vi "HEWH Adjust Gas Energy at 23 hours.vi"(0 "Full Data w/o Information Header in":dbl[][](array[numeric]) format="%#_6f", 2 "Test Start Index  (Full Index)":i32, 3 "Energy (BTU) Index":i32, 5 "error in (no error)":errorcluster) -> (14 "Qf":dbl, 15 "Start Energy (BTU-Gas)":dbl format="%#_6f", 19 "error out":errorcluster)   [LabVIEW 2020]
panel:
  out "End Energy (BTU-Gas)":dbl format="%#_11f"
  out "23 Hour Index":i32
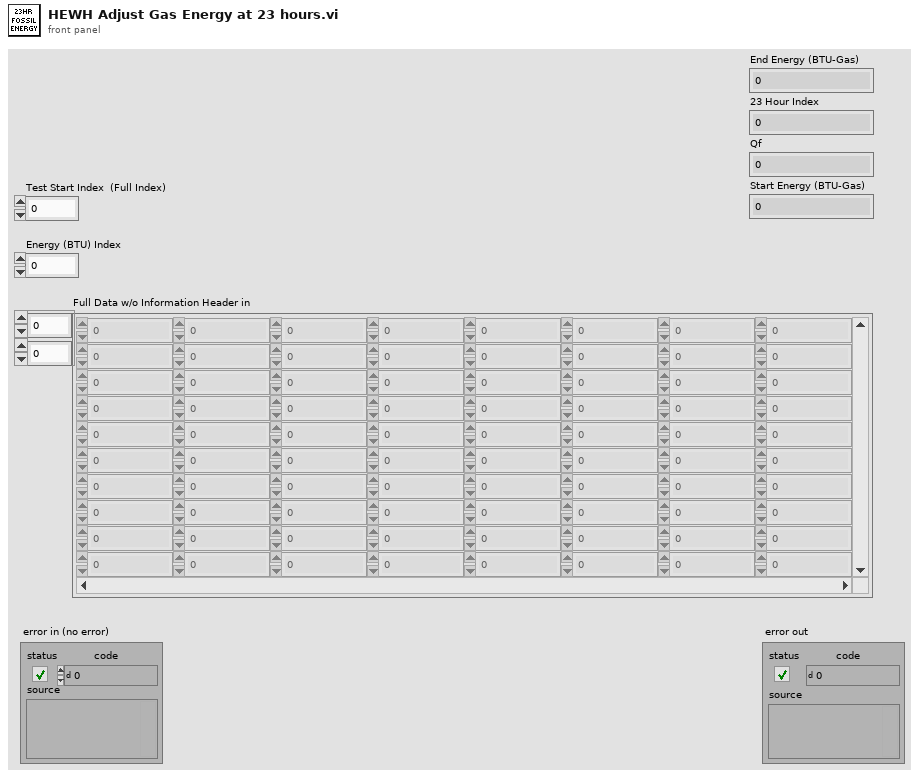
[diagram p1: front panel]
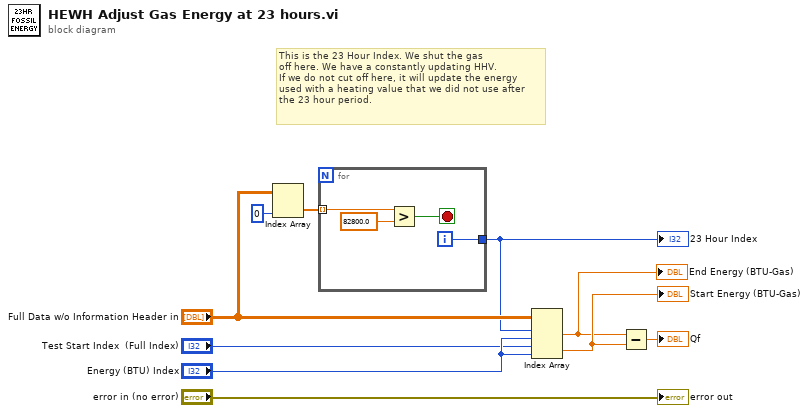
[diagram p0: block diagram]
diagram:
  # "This is the 23 Hour Index. We shut the gas\noff here. We have a constantly updating HHV. \nIf we do not cut off here, it will update the energy \nused with a heating value that we did not use after\nthe 23 hour period."
  n1 = Index Array(array="Full Data w/o Information Header in", index (col)=0 ("disabled index (col)")) -> (element=w2:dbl[])  [unwired: 1 in]
  n2 = for {
    tunnel: w2 -> [w14] mode=indexing
    tunnel: [w11] -> w1
    i -> [w11]
    stop <- w12 stop-if-true
    n3 = Greater?(x=w14, y=82800.0) -> (0:w12:bool)
  }
  "23 Hour Index" <- w1
  n4 = Index Array(array="Full Data w/o Information Header in", index (row) #1=w1, index (col) #1="Energy (BTU) Index", index (row) #2="Test Start Index  (Full Index)", index (col) #2="Energy (BTU) Index") -> (element #1=w8:dbl, element #2=w9:dbl)
  "Start Energy (BTU-Gas)" <- w9
  "End Energy (BTU-Gas)" <- w8
  n5 = Subtract(x=w8, y=w9) -> (x-y=→"Qf":dbl)
  "error out" <- "error in (no error)"
